vi "Get_Day_File_Data.vi"(4 "Averaging Time (min)":dbl=5.0, 5 "End time":timestamp, 6 "Start time":timestamp, 7 "Channel Names":string[](array[string])=["EnFlo Tun:Usonic Fixed:Velocity"], 8 "Data folder location":path) -> (0 "Files with wrong times":path[](array[path]), 1 "All Channel Names":string[](array[string]), 2 "Data":dbl[][](array[numeric]), 3 "Times":dbl[](array[numeric]))   [LabVIEW 2010]
uses:
  Anemometry/Anemometry Sub Vis/Globals/Preference_global.vi
  Anemometry/Anemometry Sub Vis/Globals/Constants_global.vi
panel:
  out "Currenly reading":path
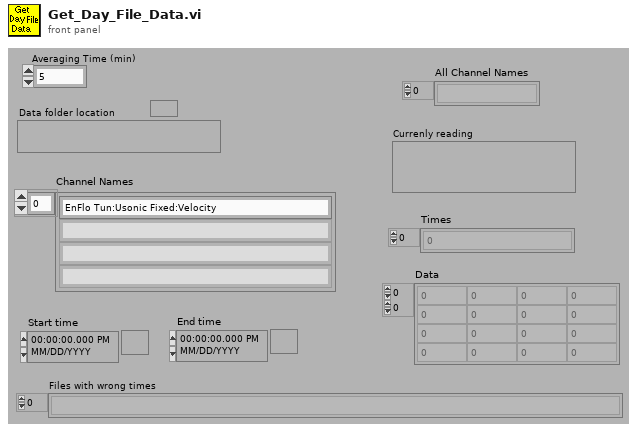
[diagram p1: front panel]
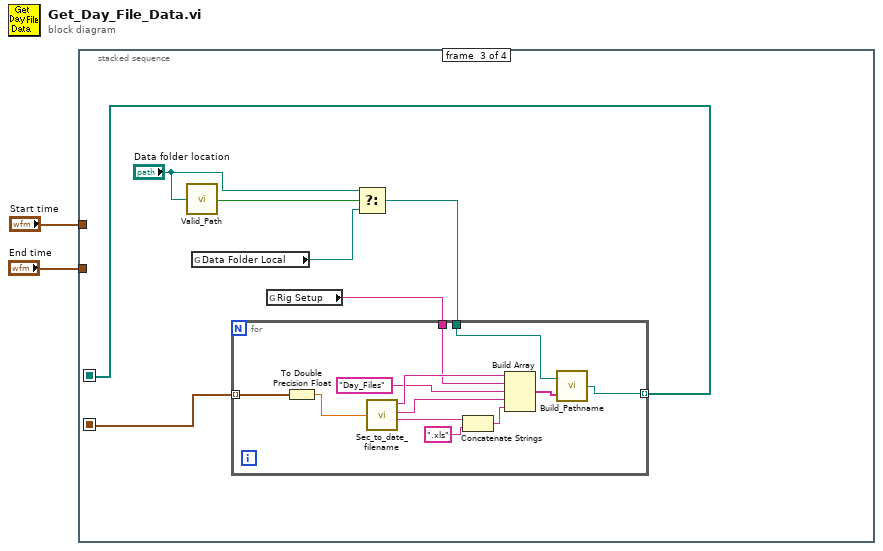
[diagram p0: block diagram]
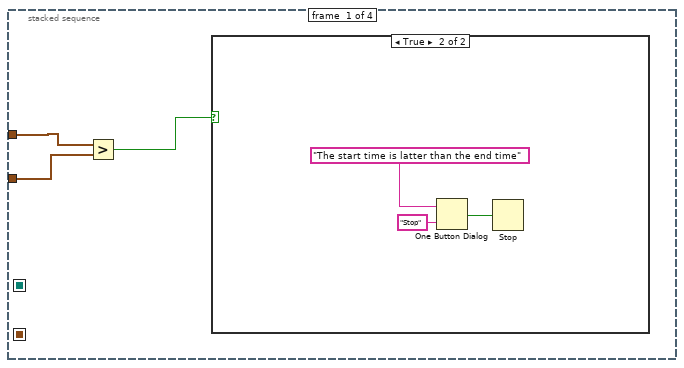
[diagram p2: hidden frame]
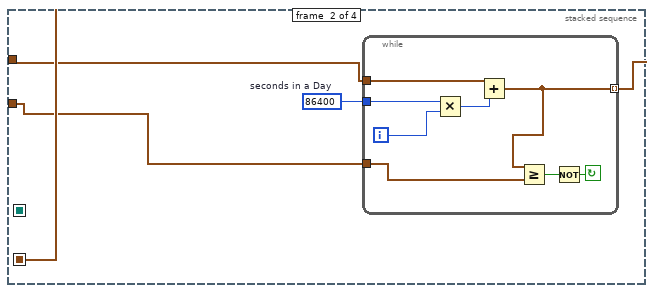
[diagram p4: hidden frame]
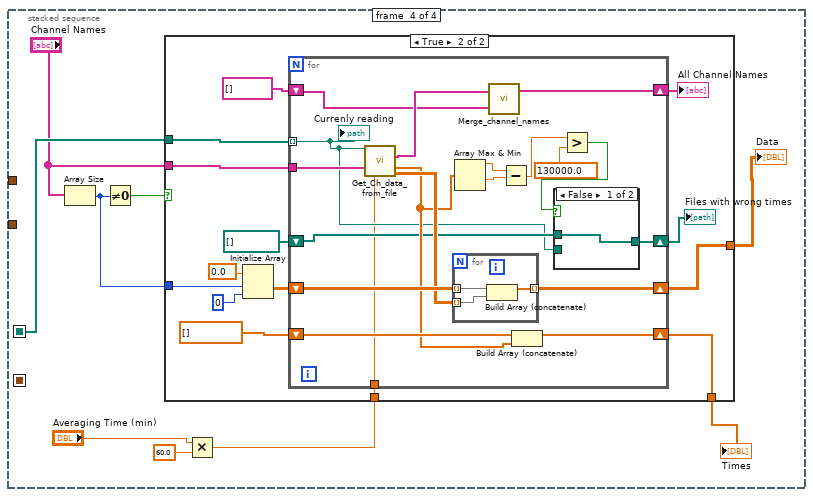
[diagram p5: hidden frame]
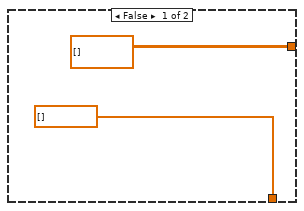
[diagram p6: hidden frame]
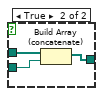
[diagram p7: hidden frame]
diagram:
  n1 = stacked-sequence {
    seq-local: [_ w12 _ _] -> [_ _ w27 _]
    seq-local: [_ _ w26 _] -> [_ _ _ w48]
    tunnel: "End time" -> [w4 w9 _ _]
    tunnel: "Start time" -> [w3 w10 _ _]
    frame #0 {
      n2 = Greater?(x=w3, y=w4) -> (0:w5:bool)
      n3 = case shown="True" w5 {
        frame False {
        }
        frame True {
          n4 = One Button Dialog(message="The start time is latter than the end time", button name ("OK")="Stop") -> (true=w7:bool)
          n5 = Stop(stop? (T)=w7) -> ()
        }
      }
    }
    frame #1 {
      w11 = u32 86400  # seconds in a Day
      n6 = while {
        tunnel: [w13] -> w12 mode=indexing
        tunnel: w9 -> [w20]
        tunnel: w10 -> [w14]
        tunnel: w11 -> [w16]
        i -> [w17]
        stop <- w18 continue-if-true
        n7 = Multiply(x=w16, y=w17) -> (x*y=w15:u32)
        n8 = Add(x=w14, y=w15) -> (x+y=w13:timestamp)
        n9 = Greater Or Equal?(x=w13, y=w20) -> (x >= y?=w19:bool)
        n10 = Not(x=w19) -> (.not. x?=w18:bool)
      }
    }
    frame #2 {
      n11 = call "Valid_Path.vi"("Filename"="Data folder location") -> ("Valid Path?"=w25:bool)
      n12 = global read "Constants_global.vi" "Data Folder Local"() -> (w23:path)
      n13 = global read "Preference_global.vi" "Rig Setup"() -> (w21:string)
      n14 = Select(t="Data folder location", s=w25, f=w23) -> (s? t:f=w22:path)
      n15 = for {
        tunnel: w27 -> [w39] mode=indexing
        tunnel: w22 -> [w32]
        tunnel: [w29] -> w26 mode=indexing
        tunnel: w21 -> [w28]
        n16 = To Double Precision Float(number=w39) -> (double precision float=w30:dbl)
        n17 = call "Sec_to_date_filename.vi"("seconds"=w30) -> ("Year"=w35:string, "Month"=w34:string, "Day"=w38:string)  [unwired: 1 out]
        n18 = Concatenate Strings(w38, ".xls" ("string")) -> (w36:string)
        n19 = Build Array(w35, w28, "Day_Files" ("Input Element"), w34, w36) -> (w31:string[])
        n20 = call "Build_Pathname.vi"("Output Array"=w31, "Pathname"=w32) -> ("Appended path"=w29:path)
      }
    }
    frame #3 {
      n21 = Array Size(array="Channel Names") -> (size(s)=w46:i32)
      n22 = Not Equal To 0?(x=w46) -> (x != 0?=w47:bool)
      n23 = Multiply(x="Averaging Time (min)", y=60.0) -> (x*y=w40:dbl)
      n24 = case shown="True" w47 {
        tunnel: w48 -> [_ w64]
        tunnel: [dbl[] [] w62] -> w44
        tunnel: [dbl[][] [] w61] -> w43
        tunnel: "Channel Names" -> [_ w59]
        tunnel: w46 -> [_ w57]
        tunnel: w40 -> [_ w51]
        frame False {
        }
        frame True {
          n25 = Initialize Array(0.0, w57, 0 ("Dimension Size")) -> (w55:dbl[][])
          n26 = for {
            tunnel: w64 -> [w66] mode=indexing
            shift-right: [w82] -> w61
            shift-left: w55 -> [w83]
            shift-right: [w81] -> w62
            shift-left: dbl[] [] -> [w80]
            shift-right: [w76] -> w52
            shift-left: string[] [] ("Merged Channels") -> [w77]
            tunnel: w59 -> [w75]
            shift-right: [w67] -> w53
            shift-left: path[] [] -> [w68]
            tunnel: w51 -> [w65]
            n27 = call "Get_Ch_data_from_file.vi"("Filename"=w66, "Channel names"=w75, "Averaging Time(s)"=w65) -> ("File Channels"=w78:string[], "Times"=w74:dbl[], "Ch Data"=w79:dbl[][])  [unwired: 1 in, 9 out]
            n28 = for {
              tunnel: w83 -> [w90] mode=indexing
              tunnel: [w89] -> w82 mode=indexing
              tunnel: w79 -> [w88] mode=indexing
              n29 = Build Array (concatenate)(w90, w88) -> (w89:dbl[])
            }
            n30 = Array Max & Min(array=w74) -> (max value=w73:dbl, min value=w72:dbl)  [unwired: 2 out]
            n31 = call "Merge_channel_names.vi"("Preferred Channel array"=w78, "Channel array"=w77) -> ("Merged Channels"=w76:string[])  [unwired: 2 out]
            n32 = Subtract(x=w73, y=w72) -> (x-y=w71:dbl)
            n33 = Build Array (concatenate)(w80, w74) -> (w81:dbl[])
            n34 = Greater?(x=w71, y=130000.0) -> (0:w69:bool)
            n35 = case shown="False" w69 {
              tunnel: w68 -> [w84 w87]
              tunnel: [w84 w86] -> w67
              tunnel: w66 -> [_ w85]
              frame False {
              }
              frame True {
                n36 = Build Array (concatenate)(w87, w85) -> (w86:path[])
              }
            }
            "Currenly reading" <- w66
          }
          "Files with wrong times" <- w53
          "All Channel Names" <- w52
        }
      }
      "Times" <- w44
      "Data" <- w43
    }
  }
